vi "User Actor Core Init.vi"(0 "MainUI in":refnum<class "MainUI.lvclass">, 11 "Error in":errorcluster caption="Error in (no error)") -> (4 "MainUI out":refnum<class "MainUI.lvclass">, 15 "Error out":errorcluster)   [LabVIEW 2018, in "HOG MainUI.lvlib" / "MainUI.lvclass"]
doc: "Initialize custom <B>Actor</B> resources. Typical actions:\n\n- Set ActorCore as normal window\n- Set Origin and Resize front panel\n- Center window on screen\n\nKåre Juul Kirkegaard\nHOG Svømning\n2/8 2017"
uses:
  MainUI.lvclass
  MainUI.lvclass/MainUI.ctl
  <vilib>/GPower/UI/Library/GP UI.lvlib
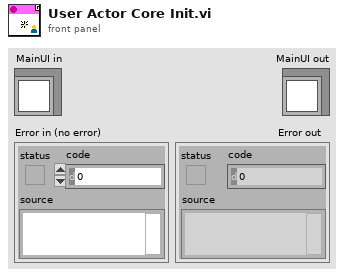
[diagram p1: front panel]
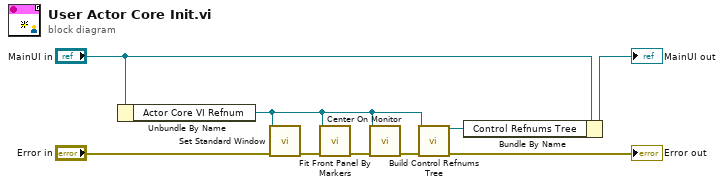
[diagram p0: block diagram]
diagram:
  n1 = Unbundle By Name("MainUI in") -> ("Actor Core VI Refnum"=w4:refnum<vi>)
  n2 = call <vilib>:"Set Standard Window.vi"("VI Refnum"=w4, "Error in"="Error in") -> ("Error out"=w9:errorcluster)  [unwired: 13 in]
  n3 = call <vilib>:"Fit Front Panel By Markers.vi"("VI Refnum"=w4, "Error in"=w9) -> ("Error out"=w8:errorcluster)  [unwired: 13 in]
  n4 = call <vilib>:"Center On Monitor.vi"("VI Refnum"=w4, "Error in"=w8) -> ("Error out"=w6:errorcluster)  [unwired: 13 in]
  n5 = call <vilib>:"Build Control Refnums Tree.vi"("VI Refnum"=w4, "Error in"=w6) -> ("Control Refnums Tree"=w1:refnum<class "Dictionary.lvclass">, "Error out"=→"Error out":errorcluster)  [unwired: 12 in]
  n6 = Bundle By Name(cluster="MainUI in", "Control Refnums Tree"=w1) -> (→"MainUI out":refnum<class "MainUI.lvclass">)
